vi "write_probes.vi"(8 "error in (no error)":errorcluster, 10 "probes":refnum<class "TempProbe.lvclass">[](array[class]), 11 "TempProbeSet in":refnum<class "TempProbeSet.lvclass">) -> (0 "error out":errorcluster, 3 "TempProbeSet out":refnum<class "TempProbeSet.lvclass">)   [LabVIEW 2010, in "TempProbeSet.lvclass"]
uses:
  TempProbeSet.lvclass
  TempProbe.lvclass
  TempProbeSet.lvclass/TempProbeSet.ctl
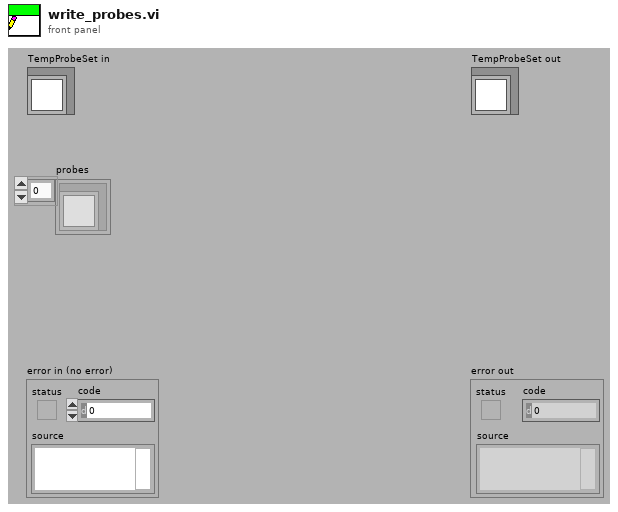
[diagram p1: front panel]
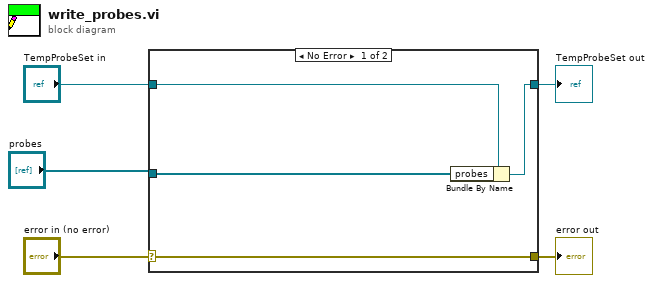
[diagram p0: block diagram]
diagram:
  n1 = case shown="No Error" "error in (no error)" {
    selector: "error in (no error)" -> [w9 w10]
    tunnel: [w9 w10] -> w4
    tunnel: [w7 w11] -> w2
    tunnel: "TempProbeSet in" -> [w8 w11]
    tunnel: "probes" -> [w6 _]
    frame No Error {
      n2 = Bundle By Name(cluster=w8, "probes"=w6) -> (w7:refnum<class "TempProbeSet.lvclass">)
    }
    frame Error {
    }
  }
  "error out" <- w4
  "TempProbeSet out" <- w2
